vi "Write Scan file path.vi"(8 "error in (no error)":errorcluster, 10 "Scan file path":path, 11 "HC-ScanParser in":refnum<class "MC-ScanParser.lvclass">) -> (0 "error out":errorcluster, 3 "HC-ScanParser out":refnum<class "MC-ScanParser.lvclass">)   [LabVIEW 2013, in "MaterialCharacterization.lvlib" / "MC-ScanParser.lvclass"]
uses:
  MC-ScanParser.lvclass
  MC-ScanParser.lvclass/MC-ScanParser.ctl
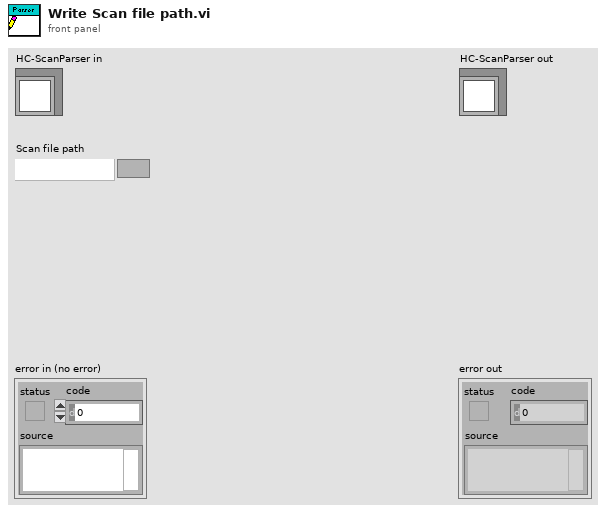
[diagram p1: front panel]
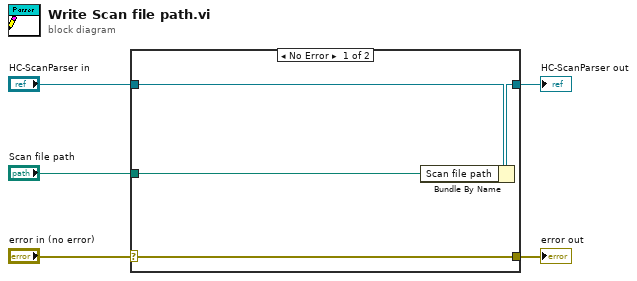
[diagram p0: block diagram]
diagram:
  n1 = case shown="No Error" "error in (no error)" {
    selector: "error in (no error)" -> [w9 w10]
    tunnel: [w9 w10] -> w4
    tunnel: [w7 w11] -> w2
    tunnel: "HC-ScanParser in" -> [w8 w11]
    tunnel: "Scan file path" -> [w6 _]
    frame No Error {
      n2 = Bundle By Name(cluster=w8, "Scan file path"=w6) -> (w7:refnum<class "MC-ScanParser.lvclass">)
    }
    frame Error {
    }
  }
  "error out" <- w4
  "HC-ScanParser out" <- w2
